vi "frez.vi"(10 "Cz":dbl, 11 "L":dbl) -> (3 "f_rez":dbl)   [LabVIEW 2020]
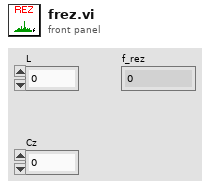
[diagram p1: front panel]
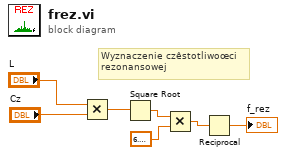
[diagram p0: block diagram]
diagram:
  # "Wyznaczenie czêstotliwoœci \nrezonansowej"
  n1 = Multiply(x="L", y="Cz") -> (x*y=w1:dbl)
  n2 = Square Root(x=w1) -> (sqrt(x)=w3:dbl)
  n3 = Multiply(x=w3, y=6.283185307179586) -> (x*y=w5:dbl)
  n4 = Reciprocal(x=w5) -> (1/x=→"f_rez":dbl)
